vi "create Snake.vi"(8 "error in (no error)":errorcluster, 10 "Starting Point":cluster{"x":u32, "y":u32}, 11 "Snake in":refnum<class "Snake.lvclass">) -> (0 "error out":errorcluster, 3 "Snake out":refnum<class "Snake.lvclass">)   [LabVIEW 2020, in "Snake.lvclass"]
uses:
  Snake.lvclass
  Snake Segment STYP.ctl
  Direction STYP.ctl
  Snake.lvclass/Snake.ctl
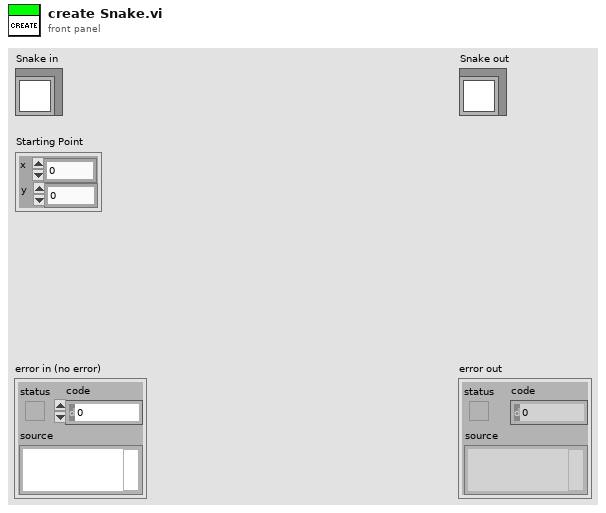
[diagram p1: front panel]
types:
  T1 = typedef "Direction STYP.ctl" = enum16{"Up", "Down", "Left", "Right"}
  T2 = typedef "Snake.lvclass/Snake Segment STYP.ctl" = cluster{"Location":cluster{"x":u32, "y":u32}, "Direction":T1}
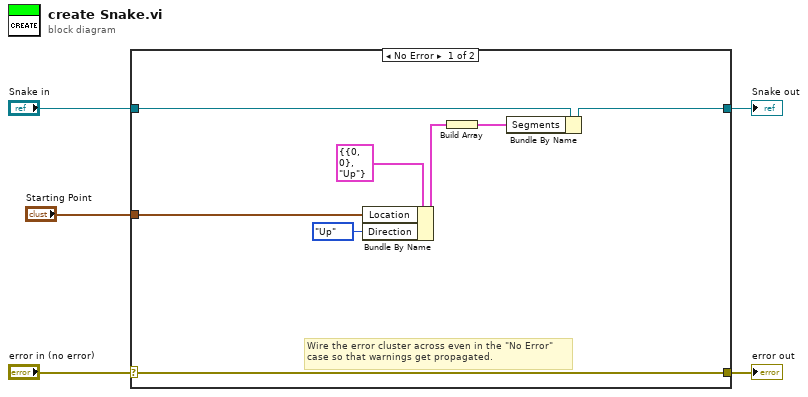
[diagram p0: block diagram]
diagram:
  n1 = case shown="No Error" "error in (no error)" {
    selector: "error in (no error)" -> [w12 w15]
    tunnel: [w12 w15] -> w4
    tunnel: [w11 w14] -> w2
    tunnel: "Snake in" -> [w13 w14]
    tunnel: "Starting Point" -> [w8 _]
    frame No Error {
      # "Wire the error cluster across even in the \"No Error\"\ncase so that warnings get propagated."
      n2 = Bundle By Name(cluster=T2 {"Location"={"x"=0, "y"=0}, "Direction"=enum."Up"} ("Snake Segment"), "Location"=w8, "Direction"=Direction_STYP."Up") -> (w7:T2)
      n3 = Build Array(w7) -> (w6:T2[])
      n4 = Bundle By Name(cluster=w13, "Segments"=w6) -> (w11:refnum<class "Snake.lvclass">)
    }
    frame Error {
    }
  }
  "error out" <- w4
  "Snake out" <- w2
